vi "Afficher_Toutes_Cdes_&_Indics.vi"() -> ()   [LabVIEW 2017, in "ALR3206T.lvlib"]
uses:
  <instrlib>/elc_2014/ALR3206T/ALR3206T.lvlib
panel:
  out "VI Ref":refnum<vi>
  out "Shown Ctls":refnum<vi>[](array[refnum])
  out "Ctl Labels":string[](array[string])=["Cluster Offset Input", "Affichage chaîne", "Affichage numérique", "CMOS (chaîne)", "Activation CMOS", "VISA Fb Error Gal", "itérations\nMain Loop", "Mémoire 1", "Mémoire 2", "Mémoire 3", "Mémoire 6", "Mémoire 4", "Mémoire 5", "Mémoire 7", "Mémoire 8", "Mémoire 9", "Mémoire 10", "Commande onglet 3", "Commande onglet 2", "VISA Error Out", "VISA Error In", "VISA Name Out", "Activation Modulation Fréquence", "Activation Modulation Amplitude", "CMOS (chaîne)", "Activation Freq Ext", "Ext.FREQ.Old"]
  out "Number Shown":i32=27
  out "error out":errorcluster
  in  "VI Name":string="IHM_R3206D.vi"
  in  "error in (no error)":errorcluster
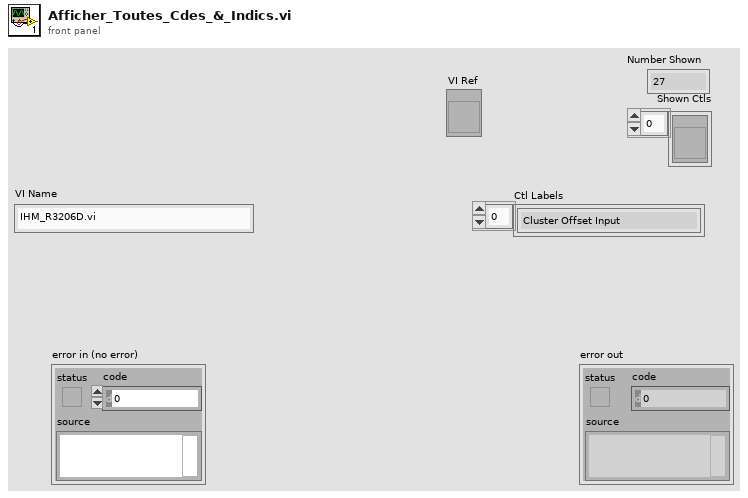
[diagram p1: front panel]
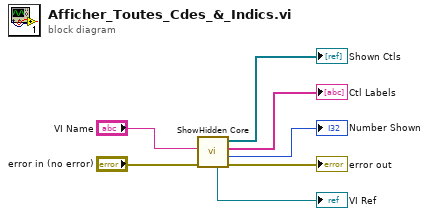
[diagram p0: block diagram]
diagram:
  n1 = call <instrlib>:"ShowHidden Core.vi"("error in (no error)"="error in (no error)", "VI Name"="VI Name") -> ("error out"=→"error out":errorcluster, "Number Shown"=→"Number Shown":i32, "Ctl Labels"=→"Ctl Labels":string[], "Shown Ctls"=→"Shown Ctls":refnum<vi>[], "VI Ref"=→"VI Ref":refnum<vi>)  [unwired: 5 in]
